vi "Frequency Response.vi"() -> ()   [LabVIEW 2020]
uses:
  <vilib>/Analysis/4window.llb/windowTd.ctl
  <vilib>/Waveform/WDTOps.llb/WDT Number of Waveform Samples DBL.vi
  <vilib>/measure/maspectr.llb/FFT Spectrum (Mag-Phase) for N Chan.vi
  <vilib>/measure/maspectr.llb/FFT Spectrum (Mag-Phase) for 1 Chan.vi
  <vilib>/Analysis/NI_AALBase.lvlib
  <vilib>/measure/NI_MAPro.lvlib
  <vilib>/Analysis/NI_AALPro.lvlib
panel:
  in  "Instrument Gain":dbl=1.0 min=0.0 max=10.0
  out "Calculating":bool
  out "Outputting":bool
  out "Waveform Graph":dynamicdata(graph)
  in  "Runtime (s)":dbl=5.0 min=0.0 max=10.0
  in  "Amplitude (Vp)":dbl=1.0 min=0.0 max=10.0
  in  "End Frequency (Hz)":dbl=100000.0 min=1.0 max=1000000.0
  in  "Start Frequency (Hz)":dbl=1000.0 min=0.0 max=1000000.0
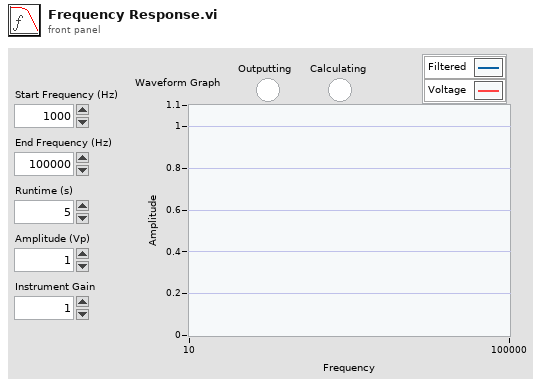
[diagram p1: front panel]
types:
  T1 = typedef "NI_AALPro.lvlib/windowTd.ctl" = u32
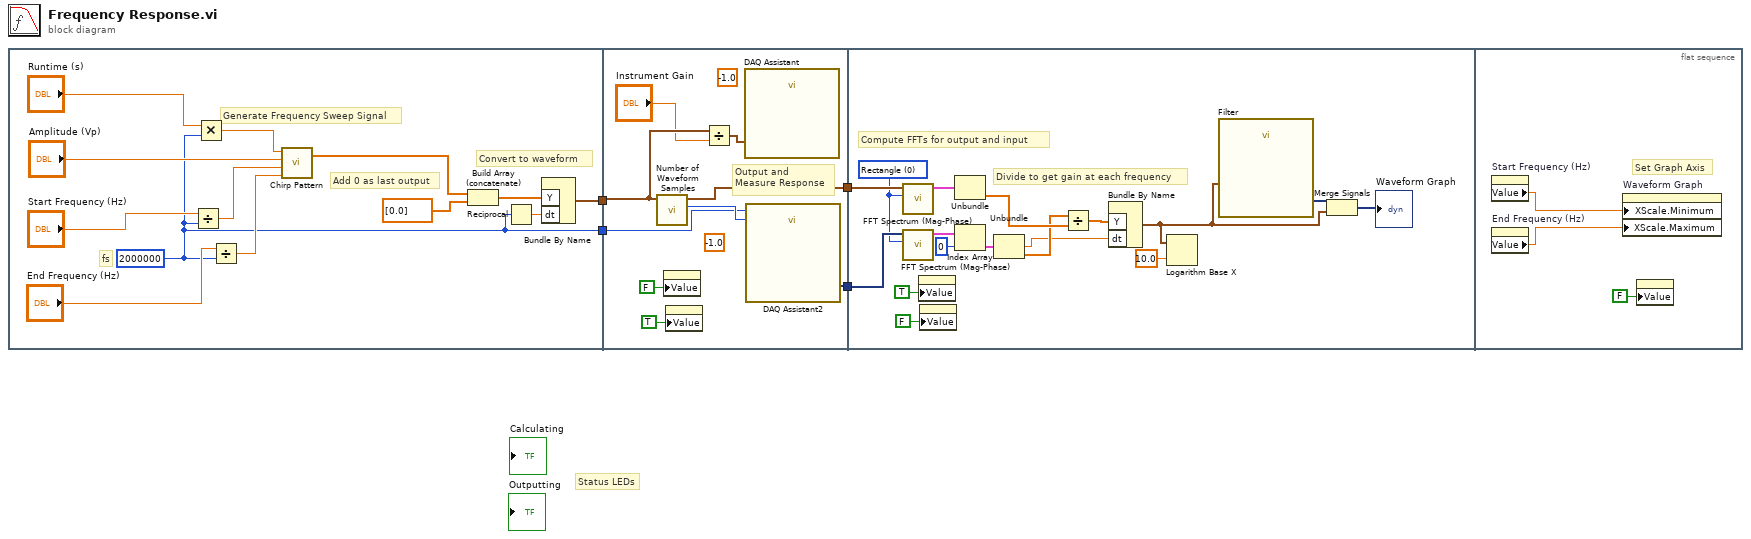
[diagram p0: block diagram]
diagram:
  # "Status LEDs"
  n1 = flat-sequence {
    tunnel: [w9] -> w4
    tunnel: [w5] -> w3
    tunnel: w4 -> [w23]
    tunnel: w3 -> [w18]
    tunnel: [w24] -> w2
    tunnel: [w20] -> w1
    tunnel: w2 -> [w43]
    tunnel: w1 -> [w42]
    frame #0 {
      w5 = 2000000
      # "Convert to waveform"
      # "Add 0 as last output"
      # "Generate Frequency Sweep Signal"
      # "fs"
      n2 = Divide(x="Start Frequency (Hz)", y=w5) -> (x/y=w14:dbl)
      n3 = Multiply(x="Runtime (s)", y=w5) -> (x*y=w10:dbl)
      n4 = Divide(x="End Frequency (Hz)", y=w5) -> (x/y=w13:dbl)
      n5 = call <vilib>:"Chirp Pattern.vi"("f2"=w13, "f1"=w14, "amplitude"="Amplitude (Vp)", "samples"=w10) -> ("Chirp Pattern"=w8:dbl[])  [unwired: 1 out]
      n6 = Build Array (concatenate)(w8, dbl[] [0.0] ("element")) -> (w6:dbl[])
      n7 = Reciprocal(x=w5) -> (1/x=w12:dbl)
      n8 = Bundle By Name("Y"=w6, "dt"=w12) -> (w9:waveform(dbl))  [unwired: 1 in]
    }
    frame #1 {
      (unwired) -1.0 ("timeout (s)")
      (unwired) -1.0 ("timeout (s)")
      # "Output and \nMeasure Response"
      n9 = call-poly <vilib>:"Number of Waveform Samples.vi"("waveform in"=w23) -> ("number of samples"=w19:i32, "waveform out"=w24:waveform(dbl))  [unwired: 8 in, 1 out]
      n10 = property on="Calculating" class="Bool (strict)"("Value"=FALSE ("Calculating")) -> ()  [unwired: 2 in, 2 out]
      n11 = property on="Outputting" class="Bool (strict)"("Value"=TRUE ("Outputting")) -> ()  [unwired: 2 in, 2 out]
      n12 = Divide(x=w23, y="Instrument Gain") -> (x/y=w21:waveform(dbl))
      n13 = call "DAQ Assistant"("data"=w21) -> ()  [unwired: 17 in, 2 out]
      n14 = call "DAQ Assistant2"("rate"=w18, "number of samples"=w19) -> ("data"=w20:dynamicdata)  [unwired: 15 in, 2 out]
    }
    frame #2 {
      w33 = T1 0 items=["Rectangle"=0, "Hanning"=1, "Hamming"=2, "Blackman-Harris"=3, "Exact Blackman"=4, "Blackman"=5, "Flat Top"=6, "4 Term B-Harris "=7, "7 Term B-Harris"=8, "Low Sidelobe"=9, "Blackman Nuttall"=11, "Triangle"=30, "Bartlett-Hanning"=31, "Bohman"=32, "Parzen"=33, "Welch"=34, "Kaiser"=60, "Dolph-Chebyshev"=61, "Gaussian"=62] ("window")
      # "Divide to get gain at each frequency"
      # "Compute FFTs for output and input"
      n15 = call-poly <vilib>:"FFT Spectrum (Mag-Phase).vi"("window"=w33, "time signal"=w43) -> ("magnitude"=w37:cluster{"f0":dbl, "df":dbl, "magnitude":dbl[]})  [unwired: 5 in, 4 out]
      n16 = call-poly <vilib>:"FFT Spectrum (Mag-Phase).vi"("window"=w33, "time signals"=w42) -> ("magnitudes"=w39:cluster{"f0":dbl, "df":dbl, "magnitude":dbl[]}[])  [unwired: 5 in, 4 out]
      n17 = property on="Calculating" class="Bool (strict)"("Value"=TRUE ("Calculating")) -> ()  [unwired: 2 in, 2 out]
      n18 = property on="Outputting" class="Bool (strict)"("Value"=FALSE ("Outputting")) -> ()  [unwired: 2 in, 2 out]
      n19 = Unbundle(w37) -> ("magnitude"=w35:dbl[])  [unwired: 2 out]
      n20 = Index Array(array=w39, index=0) -> (element=w36:cluster{"f0":dbl, "df":dbl, "magnitude":dbl[]})
      n21 = Unbundle(w36) -> ("df"=w31:dbl, "magnitude"=w34:dbl[])  [unwired: 1 out]
      n22 = Divide(x=w34, y=w35) -> (x/y=w32:dbl[])
      n23 = Bundle By Name("Y"=w32, "dt"=w31) -> (w27:waveform(dbl))  [unwired: 1 in]
      n24 = Logarithm Base X(1:10.0 ("x"), 2:w27) -> ()  [unwired: 1 out]
      n25 = call "Filter"("Signal"=w27) -> ("Filtered Signal"=w30:dynamicdata)  [unwired: 9 in, 1 out]
      n26 = Merge Signals(w30, w27) -> (→"Waveform Graph":dynamicdata)
    }
    frame #3 {
      # "Set Graph Axis"
      n27 = property on="Start Frequency (Hz)" class="DigNum (strict)"() -> ("Value"=w45:dbl)  [unwired: 2 in, 2 out]
      n28 = property on="End Frequency (Hz)" class="DigNum (strict)"() -> ("Value"=w44:dbl)  [unwired: 2 in, 2 out]
      n29 = property on="Waveform Graph" class="WFGraph (strict)"("XScale.Minimum"=w45, "XScale.Maximum"=w44) -> ()  [unwired: 2 in, 2 out]
      n30 = property on="Calculating" class="Bool (strict)"("Value"=FALSE ("Calculating")) -> ()  [unwired: 2 in, 2 out]
    }
  }
